vi "RT_TVAr_i (SubVI).vi"(0 "roll1":dbl, 7 "Act315_Act225":dbl[](array[numeric])) -> (4 "TVA_p/TVA_y":dbl[](array[numeric]))   [LabVIEW 2017]
panel:
  out "TVA_p":dbl
  out "TVA_y":dbl
  out "Act225":dbl
  out "Act315":dbl
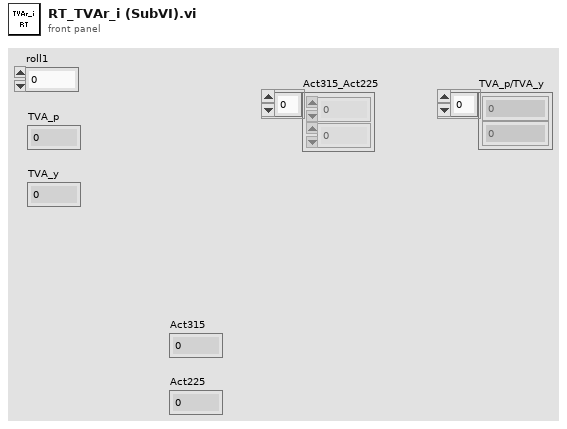
[diagram p1: front panel]
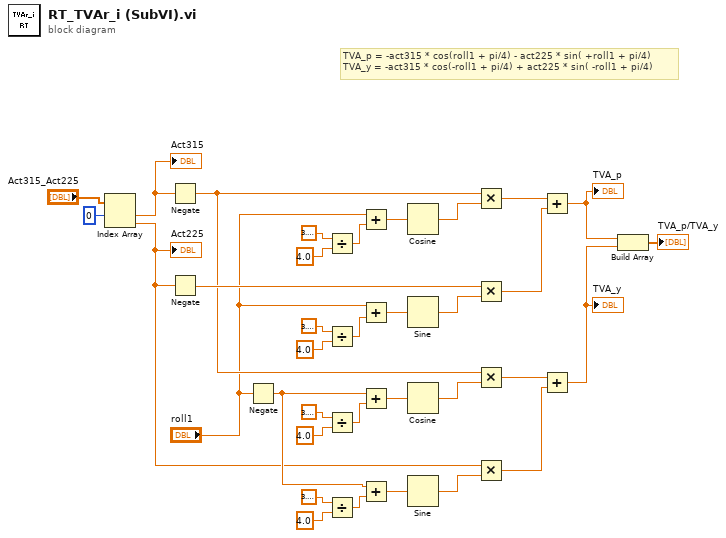
[diagram p0: block diagram]
diagram:
  # "TVA_p = -act315 * cos(roll1 + pi/4) - act225 * sin( +roll1 + pi/4)\nTVA_y = -act315 * cos(-roll1 + pi/4) + act225 * sin( -roll1 + pi/4)"
  n1 = Index Array(array="Act315_Act225", index #1=0 ("index")) -> (element #1=w30:dbl, element #2=w3:dbl)  [unwired: 1 in]
  "Act315" <- w30
  "Act225" <- w3
  n2 = Negate(x=w30) -> (-x=w7:dbl)
  n3 = Negate(x=w3) -> (-x=w23:dbl)
  n4 = Negate(x="roll1") -> (-x=w4:dbl)
  n5 = Divide(x=3.141592653589793, y=4.0) -> (x/y=w31:dbl)
  n6 = Divide(x=3.141592653589793, y=4.0) -> (x/y=w26:dbl)
  n7 = Divide(x=3.141592653589793, y=4.0) -> (x/y=w9:dbl)
  n8 = Divide(x=3.141592653589793, y=4.0) -> (x/y=w13:dbl)
  n9 = Add(x="roll1", y=w31) -> (x+y=w28:dbl)
  n10 = Add(x="roll1", y=w26) -> (x+y=w22:dbl)
  n11 = Add(x=w4, y=w9) -> (x+y=w11:dbl)
  n12 = Add(x=w4, y=w13) -> (x+y=w16:dbl)
  n13 = Cosine(x=w28) -> (cos(x)=w29:dbl)
  n14 = Sine(x=w22) -> (sin(x)=w21:dbl)
  n15 = Cosine(x=w11) -> (cos(x)=w10:dbl)
  n16 = Sine(x=w16) -> (sin(x)=w17:dbl)
  n17 = Multiply(x=w7, y=w29) -> (x*y=w27:dbl)
  n18 = Multiply(x=w23, y=w21) -> (x*y=w20:dbl)
  n19 = Multiply(x=w7, y=w10) -> (x*y=w12:dbl)
  n20 = Multiply(x=w3, y=w17) -> (x*y=w18:dbl)
  n21 = Add(x=w27, y=w20) -> (x+y=w19:dbl)
  "TVA_p" <- w19
  n22 = Add(x=w12, y=w18) -> (x+y=w2:dbl)
  "TVA_y" <- w2
  n23 = Build Array(w19, w2) -> (→"TVA_p/TVA_y":dbl[])
